vi "Filter And Analyze.vi"(10 "Y Resolution":i32, 11 "Refnum in":T1) -> (0 "Number of Particles":i32, 1 "Particle Reports (Pixels)":T3(array[cluster]) {"Orientation" format="%.2f"; "Dimensions"."Height" format="%.2f"; "Dimensions"."Width" format="%.2f"; "Center of Mass"."Y" format="%.2f"; "Center of Mass"."X" format="%.2f"; "Bounding Rect"."Bottom" format="%.2f"; "Bounding Rect"."Right" format="%.2f"; "Bounding Rect"."Top" format="%.2f"; "Bounding Rect"."Left" format="%.2f"; "Number of Holes" format="%.2f"; "Area" format="%.2f"}, 2 "Empty Array":T2(array[cluster]), 3 "Filtered Array":T2(array[cluster]))   [LabVIEW 2012]
uses:
  <vilib>/vision/Image Controls.llb/IMAQ Image.ctl
  <vilib>/vision/NI_Vision_Development_Module.lvlib
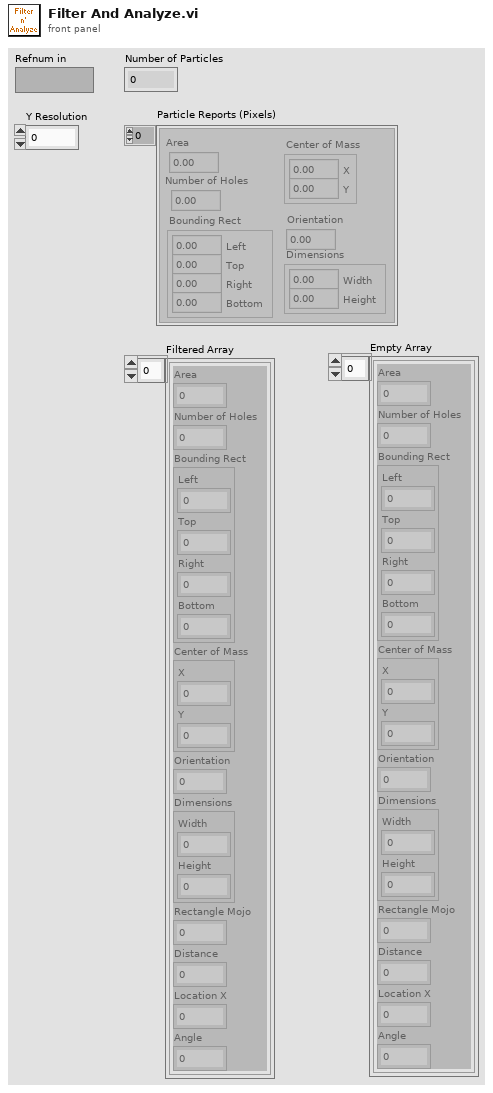
[diagram p1: front panel]
types:
  T1 = typedef "IMAQ Image.ctl" = refnum<image>
  T2 = cluster{"Area":dbl, "Number of Holes":dbl, "Bounding Rect":cluster{"Left":dbl, "Top":dbl, "Right":dbl, "Bottom":dbl}, "Center of Mass":cluster{"X":dbl, "Y":dbl}, "Orientation":dbl, "Dimensions":cluster{"Width":dbl, "Height":dbl}, "Rectangle Mojo":dbl, "Distance":dbl, "Location X":dbl, "Angle":dbl}[]
  T3 = cluster{"Area":dbl, "Number of Holes":dbl, "Bounding Rect":cluster{"Left":dbl, "Top":dbl, "Right":dbl, "Bottom":dbl}, "Center of Mass":cluster{"X":dbl, "Y":dbl}, "Orientation":dbl, "Dimensions":cluster{"Width":dbl, "Height":dbl}}[]
  T4 = cluster{"Area":dbl, "Number of Holes":dbl, "Bounding Rect":cluster{"Left":dbl, "Top":dbl, "Right":dbl, "Bottom":dbl}, "Center of Mass":cluster{"X":dbl, "Y":dbl}, "Orientation":dbl, "Dimensions":cluster{"Width":dbl, "Height":dbl}, "Rectangle Mojo":dbl, "Distance":dbl, "Location X":dbl, "Angle":dbl}
  T5 = typedef "Particle Parameters" = i32
  T6 = cluster{"Measurement Parameter":T5, "Range Lower Value":dbl, "Range Upper Value":dbl, "Range":bool, "Measurement Type":bool}[]
  T7 = typedef "Image Type" = u32
  T8 = cluster{"Left":dbl, "Top":dbl, "Right":dbl, "Bottom":dbl}
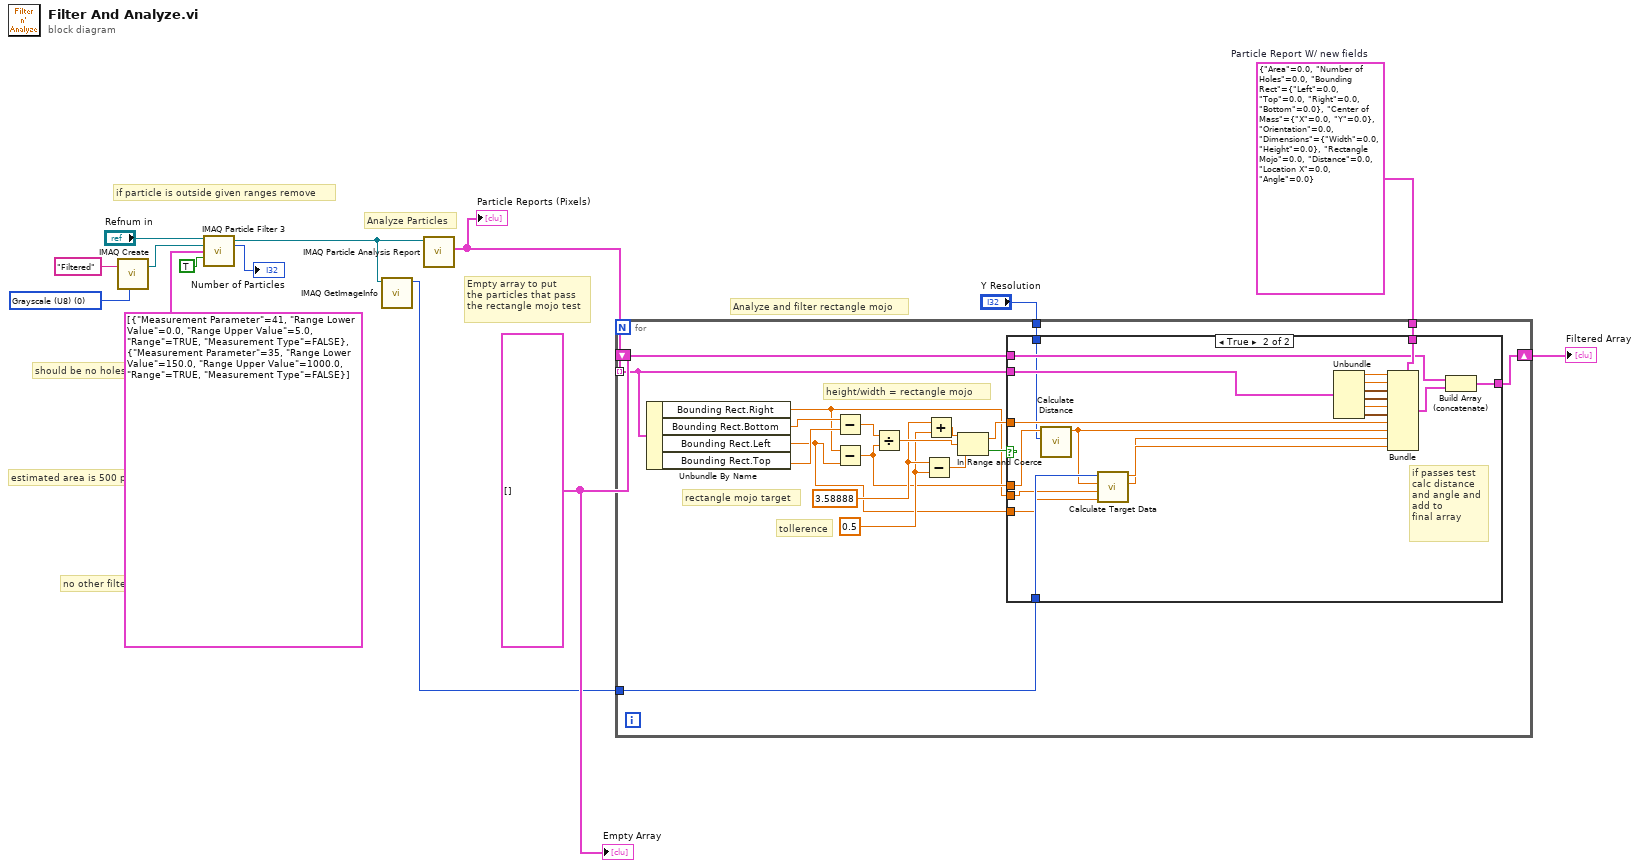
[diagram p0: block diagram]
diagram:
  w13 = T2 []
  w10 = T4 {"Area"=0.0, "Number of Holes"=0.0, "Bounding Rect"={"Left"=0.0, "Top"=0.0, "Right"=0.0, "Bottom"=0.0}, "Center of Mass"={"X"=0.0, "Y"=0.0}, "Orientation"=0.0, "Dimensions"={"Width"=0.0, "Height"=0.0}, "Rectangle Mojo"=0.0, "Distance"=0.0, "Location X"=0.0, "Angle"=0.0}  # Particle Report W/ new fields
  w3 = T7 0 items=["Grayscale (U8)", "Grayscale (I16)", "Grayscale (SGL)", "Complex (CSG)", "RGB (U32)", "HSL (U32)", "RGB (U64)", "Grayscale (U16)"] ("Image Type")
  # "Empty array to put\nthe particles that pass\nthe rectangle mojo test"
  # "Analyze and filter rectangle mojo"
  # "Analyze Particles"
  # "no other filter"
  # "should be no holes"
  # "if particle is outside given ranges remove"
  # "estimated area is 500 px"
  n1 = call "IMAQ Create"("Image Name"="Filtered", "Image Type"=w3) -> ("New Image"=w5:T1)  [unwired: 3 in, 1 out]
  n2 = call "IMAQ Particle Filter 3"("Image Src"="Refnum in", "Image Dst"=w5, "Selection Values"=T6 [{"Measurement Parameter"=41, "Range Lower Value"=0.0, "Range Upper Value"=5.0, "Range"=TRUE, "Measurement Type"=FALSE}, {"Measurement Parameter"=35, "Range Lower Value"=150.0, "Range Upper Value"=1000.0, "Range"=TRUE, "Measurement Type"=FALSE}], "Keep/Remove Particles (F)"=TRUE) -> ("Image Dst Out"=w2:T1, "Number of Particles"=→"Number of Particles":i32)  [unwired: 9 in, 1 out]
  n3 = call "IMAQ GetImageInfo"("Image"=w2) -> ("X Resolution"=w1:i32)  [unwired: 3 in, 7 out]
  n4 = call "IMAQ Particle Analysis Report"("Image"=w2) -> ("Particle Reports (Pixels)"=w9:T3)  [unwired: 5 in, 5 out]
  "Particle Reports (Pixels)" <- w9
  n5 = for {
    tunnel: w9 -> [w24] mode=indexing
    tunnel: w10 -> [w23]
    tunnel: "Y Resolution" -> [w20]
    shift-right: [w19] -> w14
    shift-left: w13 -> [w18]
    tunnel: w1 -> [w17]
    w26 = 0.5 ("upper limit")
    w27 = 3.58888 ("upper limit")
    # "tollerence"
    # "rectangle mojo target"
    # "height/width = rectangle mojo"
    n6 = Unbundle By Name(w24) -> ("Bounding Rect.Right"=w16:dbl, "Bounding Rect.Bottom"=w33:dbl, "Bounding Rect.Left"=w15:dbl, "Bounding Rect.Top"=w32:dbl)
    n7 = Subtract(x=w33, y=w32) -> (x-y=w31:dbl)
    n8 = Subtract(x=w16, y=w15) -> (x-y=w21:dbl)
    n9 = Divide(x=w31, y=w21) -> (x/y=w30:dbl)
    n10 = Subtract(x=w27, y=w26) -> (x-y=w28:dbl)
    n11 = Add(x=w27, y=w26) -> (x+y=w29:dbl)
    n12 = In Range and Coerce(upper limit=w29, x=w30, lower limit=w28) -> (coerced(x)=w22:dbl, In Range?=w25:bool)
    n13 = case shown="True" w25 {
      tunnel: w24 -> [_ w52]
      tunnel: [w34 w54] -> w19
      tunnel: w18 -> [w34 w43]
      tunnel: w23 -> [_ w53]
      tunnel: w22 -> [_ w45]
      tunnel: w21 -> [_ w42]
      tunnel: w20 -> [_ w41]
      tunnel: w17 -> [_ w38]
      tunnel: w16 -> [_ w36]
      tunnel: w15 -> [_ w35]
      frame False {
        # "if fails test don't add\nto final array"
      }
      frame True {
        # "if passes test\ncalc distance\nand angle and\nadd to\nfinal array"
        n14 = call "Calculate Distance.vi"("Y Resolution"=w41, "Target Height (px)"=w42) -> ("Distance"=w37:dbl)  [unwired: 9 in]
        n15 = call "Calculate Target Data.vi"("Rect Left"=w35, "Rect Right"=w36, "Distance to Target (ft)"=w37, "Image Width (px)"=w38) -> ("X Location"=w39:dbl, "Angle"=w40:dbl)  [unwired: 6 in]
        n16 = Unbundle(w52) -> ("Area"=w51:dbl, "Number of Holes"=w50:dbl, "Bounding Rect"=w49:T8, "Center of Mass"=w48:cluster{"X":dbl, "Y":dbl}, "Orientation"=w47:dbl, "Dimensions"=w46:cluster{"Width":dbl, "Height":dbl})
        n17 = Bundle(cluster=w53, "Area"=w51, "Number of Holes"=w50, "Bounding Rect"=w49, "Center of Mass"=w48, "Orientation"=w47, "Dimensions"=w46, "Rectangle Mojo"=w45, "Distance"=w37, "Location X"=w39, "Angle"=w40) -> (w44:T4)
        n18 = Build Array (concatenate)(w43, w44) -> (w54:T2)
      }
    }
  }
  "Filtered Array" <- w14
  "Empty Array" <- w13
